vi "Build Output Directory.vi"(8 "error in (no error)":errorcluster, 11 "Parse Presentation in":refnum<class "Parse Presentation.lvclass">) -> (0 "error out":errorcluster, 3 "Parse Presentation out":refnum<class "Parse Presentation.lvclass">)   [LabVIEW 2015, in "Parse Presentation.lvclass"]
uses:
  Parse Presentation.lvclass
  Parse Presentation.lvclass/Parse Presentation.ctl
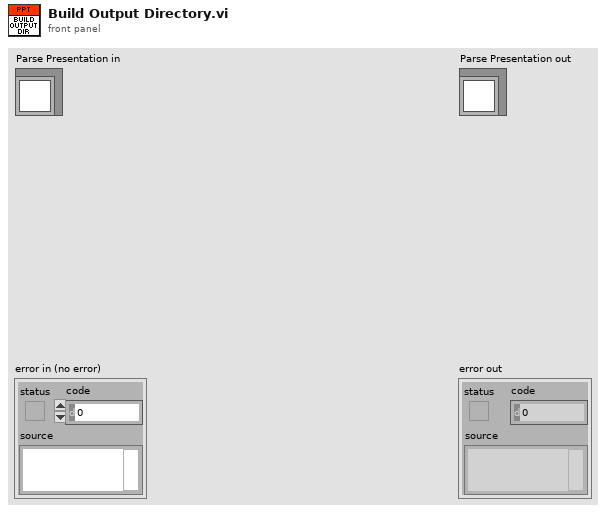
[diagram p1: front panel]
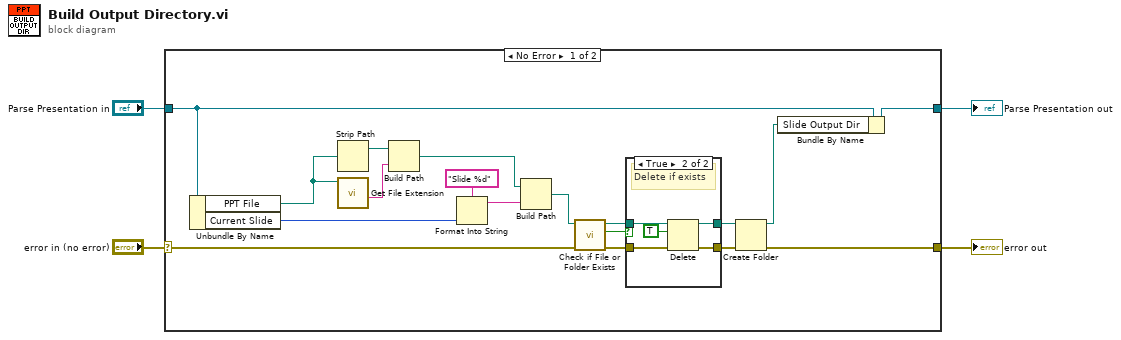
[diagram p0: block diagram]
diagram:
  n1 = case shown="No Error" "error in (no error)" {
    selector: "error in (no error)" -> [w9 w31]
    tunnel: [w8 w31] -> w3
    tunnel: [w6 w30] -> w1
    tunnel: "Parse Presentation in" -> [w10 w30]
    frame No Error {
      n2 = Unbundle By Name(w10) -> ("PPT File"=w7:path, "Current Slide"=w12:i32)
      n3 = Strip Path(path=w7) -> (stripped path=w14:path)  [unwired: 1 out]
      n4 = call <vilib>:"Get File Extension.vi"("file"=w7) -> ("filename without extension"=w15:string)  [unwired: 6 in, 4 out]
      n5 = Build Path(base path=w14, name or relative path=w15) -> (appended path=w16:path)
      n6 = Format Into String(format string="Slide %d", w12) -> (resulting string=w13:string)  [unwired: 2 in, 1 out]
      n7 = Build Path(base path=w16, name or relative path=w13) -> (appended path=w22:path)
      n8 = call <vilib>:"Check if File or Folder Exists.vi"("error in (no error)"=w9, "path"=w22) -> ("error out"=w17:errorcluster, "file or folder exists?"=w18:bool, "dup path"=w19:path)  [unwired: 7 in]
      n9 = case shown="True" w18 {
        tunnel: w19 -> [w23 w29]
        tunnel: w17 -> [w24 w28]
        tunnel: [w24 w27] -> w21
        tunnel: [w23 w26] -> w20
        frame False {
        }
        frame True {
          # "Delete if exists"
          n10 = Delete(path (use dialog)=w29, entire hierarchy (F)=TRUE, error in=w28) -> (deleted path=w26:path, error out=w27:errorcluster)  [unwired: 2 in, 1 out]
        }
      }
      n11 = Create Folder(path (use dialog)=w20, error in=w21) -> (created path=w5:path, error out=w8:errorcluster)  [unwired: 1 in, 1 out]
      n12 = Bundle By Name(cluster=w10, "Slide Output Dir"=w5) -> (w6:refnum<class "Parse Presentation.lvclass">)
    }
    frame Error {
    }
  }
  "error out" <- w3
  "Parse Presentation out" <- w1
